vi "SRS_QCM_SubVI.vi"(0 "VISA Refnum in":refnum<visa-resource-name>, 1 "first iteration?":bool, 5 "Frequency out 3":dbl, 7 "Boolean 2":bool, 9 "Gate time":u16(ring)=1 items=["0.1 seconds", "1.0 seconds", "10.0 seconds"], 11 "error in (no error)":errorcluster) -> (3 "Frequency out 2":dbl, 4 "Cluster":T3, 6 "Frequency out":dbl format="%#_8g", 8 "Cluster 2":T2, 10 "M":string, 13 "MR":string, 14 "F":string, 15 "M,F,MR output cluster":T1)   [LabVIEW 2014]
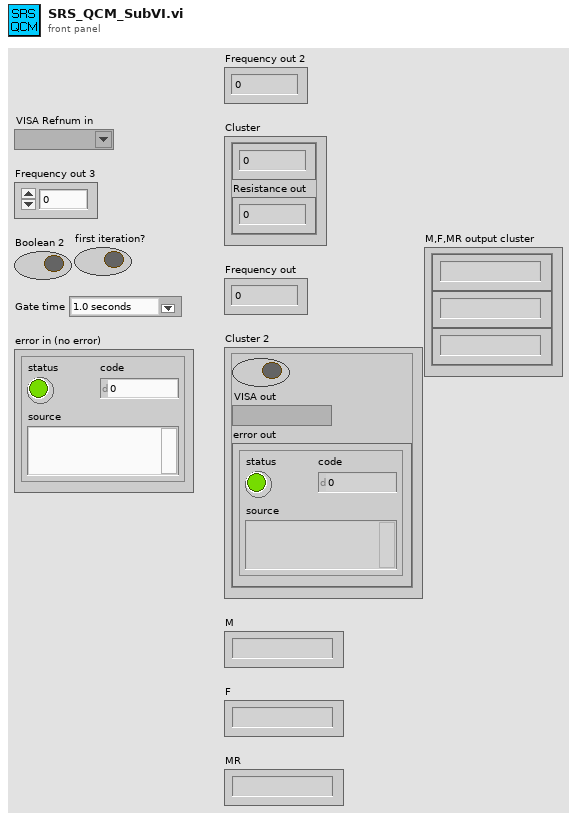
[diagram p1: front panel]
types:
  T1 = cluster{"String":string, "String":string, "String":string}
  T2 = cluster{"Boolean":bool, "VISA out":refnum<visa-resource-name>, "error out":errorcluster}
  T3 = cluster{"Numeric Control":dbl, "Resistance out":dbl}
  T4 = cluster{"Boolean 2":bool, "VISA out":refnum<visa-resource-name>, "error out":errorcluster}
  T5 = cluster{dbl, "Frequency out":dbl, "Resistance out":dbl}
  T6 = cluster{string, "Frequency out":string, "Resistance out":string}
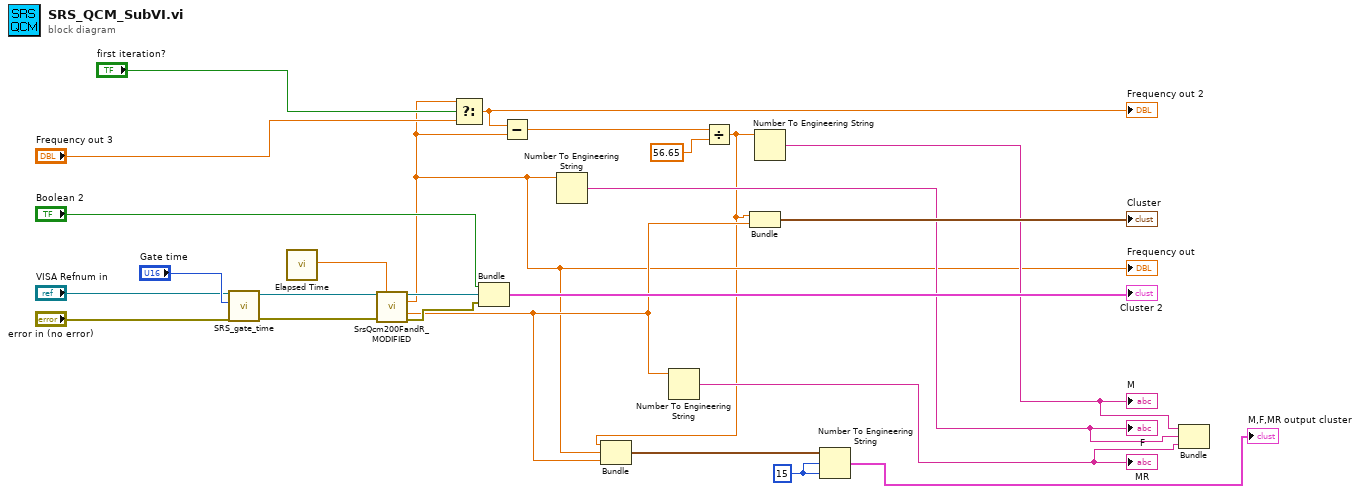
[diagram p0: block diagram]
diagram:
  w3 = i16 15 ("width (-)")
  n1 = call "SRS_gate_time.vi"("error in"="error in (no error)", "Gate time"="Gate time", "VISA in"="VISA Refnum in") -> ("error out"=w23:errorcluster, "VISA out"=w22:refnum<visa-resource-name>)  [unwired: 7 in]
  n2 = call "Elapsed Time"() -> ("Elapsed Time (s)"=w13:dbl)  [unwired: 12 in, 7 out]
  n3 = call "SrsQcm200FandR_MODIFIED.vi"("VISA in"=w22, "Reference time in"=w13, "error in (no error)"=w23) -> ("VISA out"=w15:refnum<visa-resource-name>, "Frequency out"=w2:dbl, "Resistance out"=w6:dbl, "error out"=w14:errorcluster)  [unwired: 6 in, 3 out]
  "Frequency out" <- w2
  n4 = Select(t=w2, s="first iteration?", f="Frequency out 3") -> (s? t:f=w19:dbl)
  "Frequency out 2" <- w19
  n5 = Bundle("Boolean 2"="Boolean 2", "VISA out"=w15, "error out"=w14) -> (→"Cluster 2":T4)  [unwired: 1 in]
  n6 = Subtract(x=w19, y=w2) -> (x-y=w17:dbl)
  n7 = Number To Engineering String(4:w2) -> (0:w7:string)  [unwired: 3 in]
  "F" <- w7
  n8 = Number To Engineering String(4:w6) -> (0:w8:string)  [unwired: 3 in]
  "MR" <- w8
  n9 = Divide(x=w17, y=56.65) -> (x/y=w1:dbl)
  n10 = Bundle(w1, "Frequency out"=w2, "Resistance out"=w6) -> (w5:T5)  [unwired: 1 in]
  n11 = Bundle(w1, "Resistance out"=w6) -> (→"Cluster":cluster{dbl, "Resistance out":dbl})  [unwired: 1 in]
  n12 = Number To Engineering String(4:w1) -> (0:w9:string)  [unwired: 3 in]
  "M" <- w9
  n13 = Number To Engineering String(2:w3, 3:w3, 4:w5) -> (0:→"M,F,MR output cluster":T6)  [unwired: 1 in]
  n14 = Bundle(w9, w7, w8) -> ()  [unwired: 1 in, 1 out]
